vi "Register Kernel Event.vi"(8 "Error In":errorcluster, 9 "Kernel Handle":T3, 10 "User Event":refnum<user-event>, 11 "Device ID":T2) -> (0 "Error Out":errorcluster, 1 "User Event Out":T1, 2 "Kernel Handle Out":T3, 3 "Device ID Out":T2)   [LabVIEW 2012]
doc: "Registers a kernel user event using a Boolean Labview User Event. Once a kernel has been registered with a Labview User Event, it can be called asynchronously (non-blocking) to allow other tasks to be performed by the program including user inputs to the front panel."
uses:
  Non-User VIs/Controls/Kernel Handle.ctl
  Non-User VIs/Controls/Device ID.ctl
  Non-User VIs/Controls/User Event.ctl
  Non-User VIs/Error Checking/Add Error Functional Global.vi
  OpenCLV x64.lvlib
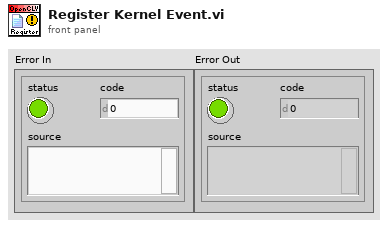
[diagram p1: front panel]
types:
  T1 = typedef "OpenCLV x64.lvlib/User Event.ctl" = refnum<user-event>
  T2 = typedef "OpenCLV x64.lvlib/Device ID.ctl" = u64
  T3 = typedef "OpenCLV x64.lvlib/Kernel Handle.ctl" = u64
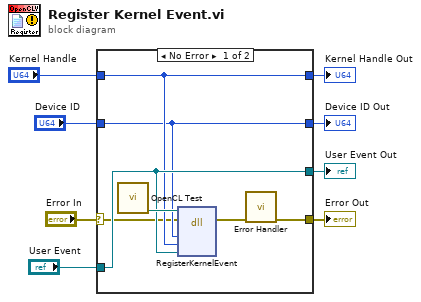
[diagram p0: block diagram]
diagram:
  n1 = case shown="No Error" "Error In" {
    selector: "Error In" -> [w9 w19]
    tunnel: [w10 w19] -> w7
    tunnel: "Kernel Handle" -> [w13 w17]
    tunnel: "User Event" -> [w14 w18]
    tunnel: [w13 w17] -> w5
    tunnel: [w14 w18] -> w1
    tunnel: "Device ID" -> [w12 w16]
    tunnel: [w12 w16] -> w3
    frame No Error {
      n2 = call "OpenCL Test.vi"() -> ("DLL To Use"=w15:path)  [unwired: 11 in]
      n3 = dll-call lib="D:/OpenCLV/trunk/OpenCLV_x64_1.0/OpenCLV_x64.dll" fn="RegisterKernelEvent"(path in=w15, error in=w9, "Device"=w12, "Kernel"=w13, "Labview Event"=w14) -> (error out=w11:errorcluster)  [unwired: 5 in, 1 out]
      n4 = call-poly "Error Handler.vi"("Error In"=w11) -> ("Error Out"=w10:errorcluster)  [unwired: 10 in]
    }
    frame Error {
    }
  }
  "Error Out" <- w7
  "Kernel Handle Out" <- w5
  "Device ID Out" <- w3
  "User Event Out" <- w1
